vi "例8.9 连续输出(允许重生成)2.vi"() -> ()   [LabVIEW 2017]
uses:
  <vilib>/measure/NI_MABase.lvlib
panel:
  in  "signal type":T1(ring) caption="信号类型"
  in  "毫秒倍数":u32=150
  in  "stop (F)":bool caption="停止(F)"
  in  "sampling info":cluster{"Fs":dbl, "#s":dbl}={"Fs"=1000.0, "#s"=150.0} caption="采样信息" {"Fs" format="%.2p"}
  in  "amplitude":dbl=1.0 caption="幅值" format="%0.2p"
  in  "frequency":dbl=10.0 caption="频率" format="%0.2p"
  out "波形图":waveform(dbl)(graph)
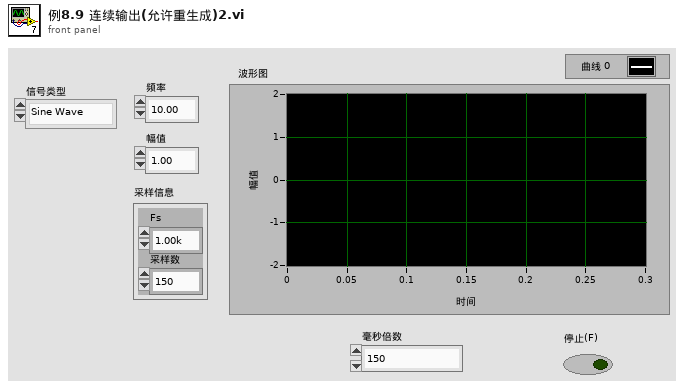
[diagram p1: front panel]
types:
  T1 = enum16{"Sine Wave", "Triangle Wave", "Square Wave", "Sawtooth Wave"}
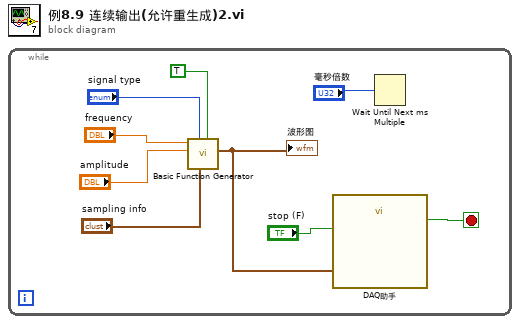
[diagram p0: block diagram]
diagram:
  n1 = while {
    stop <- w8 stop-if-true
    n2 = call <vilib>:"Basic Function Generator.vi"("reset signal"=TRUE, "sampling info"="sampling info", "signal type"="signal type", "amplitude"="amplitude", "frequency"="frequency") -> ("signal out"=w3:waveform(dbl))  [unwired: 4 in, 2 out]
    "波形图" <- w3
    n3 = call "DAQ助手"("data"=w3, "stop (F)"="stop (F)") -> ("stopped"=w8:bool)  [unwired: 15 in, 2 out]
    n4 = Wait Until Next ms Multiple(millisecond multiple="毫秒倍数") -> ()  [unwired: 1 out]
  }
